vi "Radians to Degrees.vi"(11 "Radians":dbl) -> (3 "Degrees":dbl)   [LabVIEW 2014]
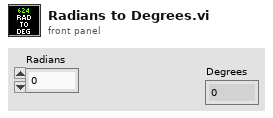
[diagram p1: front panel]
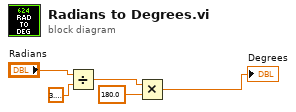
[diagram p0: block diagram]
diagram:
  n1 = Divide(x="Radians", y=3.141592653589793) -> (x/y=w3:dbl)
  n2 = Multiply(x=w3, y=180.0) -> (x*y=→"Degrees":dbl)
